vi "Stop.vi"(8 "error in (no error)":errorcluster, 11 "Analog Input in":refnum<class "Analog Input.lvclass">) -> (0 "error out":errorcluster, 3 "connection ID":i32)   [LabVIEW 2009, in "MicroDAQ.lvlib" / "Analog Input.lvclass"]
doc: "Stops acquisition and clears channel configuration on device."
uses:
  <instrlib>/MicroDAQ/Channel/Analog Input/Analog Input.lvclass
  <instrlib>/MicroDAQ/Mlink library wraper/mlink.lvlib
  <instrlib>/MicroDAQ/Channel/Channel.lvclass
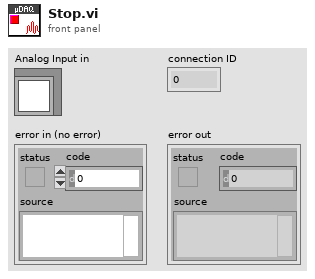
[diagram p1: front panel]
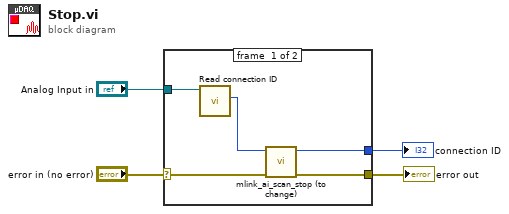
[diagram p0: block diagram]
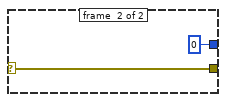
[diagram p2: hidden frame]
diagram:
  n1 = case shown="No Error" "error in (no error)" {
    selector: "error in (no error)" -> [w9 w11]
    tunnel: [w8 w11] -> w3
    tunnel: "Analog Input in" -> [w7 _]
    tunnel: [w5 0 ("connection ID out")] -> w1
    frame #0 {
      n2 = call <instrlib>:"Read connection ID.vi"("Task in"=w7) -> ("connection ID"=w6:i32)  [unwired: 9 in, 1 out]
      n3 = call <instrlib>:"mlink_ai_scan_stop (to change).vi"("error in (no error)"=w9, "connection ID"=w6) -> ("error out"=w8:errorcluster, "connection ID out"=w5:i32)  [unwired: 8 in]
    }
    frame #1 {
    }
  }
  "error out" <- w3
  "connection ID" <- w1
